vi "System Options.vi"(5 "Message Text (Empty)":string, 7 "Message (F: Off)":bool, 8 "error in (no error)":errorcluster, 9 "Beeper (T: On)":bool=TRUE, 10 "Display (T: On)":bool=TRUE, 11 "VISA resource name":refnum<visa-resource-name>) -> (0 "error out":errorcluster, 3 "VISA resource name out":refnum<visa-resource-name>)   [LabVIEW 2020, in "Agilent 34401.lvlib"]
doc: "Allows users to turn off the instrument's beeper and display."
uses:
  Agilent 34401.lvlib
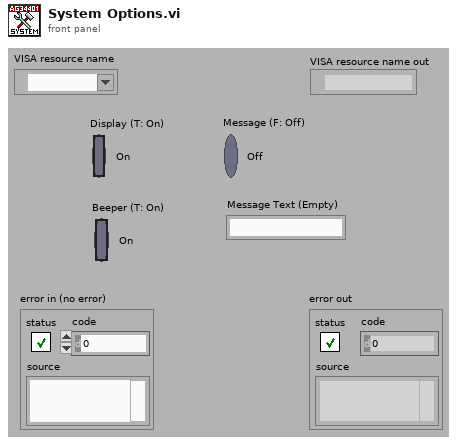
[diagram p1: front panel]
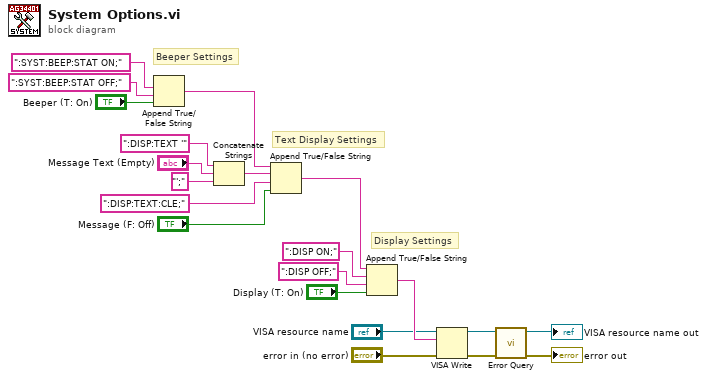
[diagram p0: block diagram]
diagram:
  # "Text Display Settings"
  # "Display Settings"
  # "Beeper Settings"
  n1 = Append True/False String(1:"Beeper (T: On)", 2:":SYST:BEEP:STAT OFF;", 3:":SYST:BEEP:STAT ON;") -> (0:w1:string)  [unwired: 1 in]
  n2 = Concatenate Strings(":DISP:TEXT '", "Message Text (Empty)", "';") -> (w5:string)
  n3 = Append True/False String(1:"Message (F: Off)", 2:":DISP:TEXT:CLE;", 3:w5, 4:w1) -> (0:w3:string)
  n4 = Append True/False String(1:"Display (T: On)", 2:":DISP OFF;", 3:":DISP ON;", 4:w3) -> (0:w15:string)
  n5 = VISA Write(VISA resource name="VISA resource name", write buffer=w15, error in (no error)="error in (no error)") -> (VISA resource name out=w12:refnum<visa-resource-name>, error out=w11:errorcluster)  [unwired: 1 out]
  n6 = call "Error Query.vi"("error in (no error)"=w11, "VISA resource name"=w12) -> ("error out"=→"error out":errorcluster, "VISA resource name out"=→"VISA resource name out":refnum<visa-resource-name>)  [unwired: 6 in, 2 out]
